vi "reallocate_pixel_mapper_arrays.vi"(7 "New pixels per spiral":T1=1 min=1 max=90000 step=1, 8 "error in":errorcluster, 9 "New image size":T2=128 items=["128x128 px"=128, "256x256 px"=256, "512x512 px"=512], 10 "Lookup arrays in":T3, 11 "Pixelhits array in":refnum<data-value>) -> (0 "error out":errorcluster, 2 "Lookup arrays out":T3, 3 "Pixelhits array out":refnum<data-value>)   [LabVIEW 2011, in "Fiberscope_library.lvlib"]
uses:
  Fiberscope_library.lvlib
  typedefs/lookup_arrays_ref_cluster.ctl
  typedefs/image_size_I32.ctl
  typedefs/pixel_per_spiral_I32.ctl
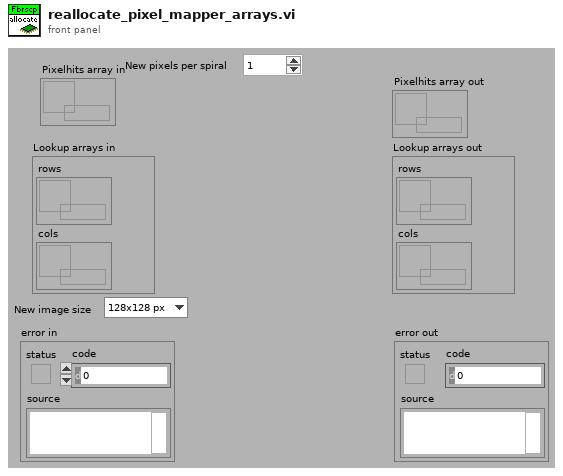
[diagram p1: front panel]
types:
  T1 = typedef "Fiberscope_library.lvlib/pixel_per_spiral_I32.ctl" = i32
  T2 = typedef "Fiberscope_library.lvlib/image_size_I32.ctl" = i32
  T3 = typedef "Fiberscope_library.lvlib/lookup_arrays_ref_cluster.ctl" = cluster{"rows":refnum<data-value>, "cols":refnum<data-value>}
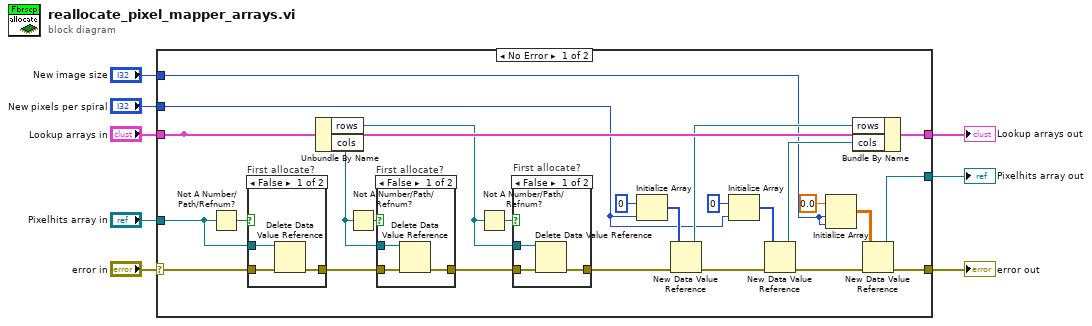
[diagram p0: block diagram]
diagram:
  n1 = case shown="No Error" "error in" {
    selector: "error in" -> [w26 w49]
    tunnel: [w19 w49] -> w7
    tunnel: [w17 w48] -> w4
    tunnel: "Pixelhits array in" -> [w16 w48]
    tunnel: [w27 w47] -> w3
    tunnel: "Lookup arrays in" -> [w28 w47]
    tunnel: "New image size" -> [w10 _]
    tunnel: "New pixels per spiral" -> [w9 _]
    frame No Error {
      n2 = Not A Number/Path/Refnum?(number/path/refnum=w16) -> (NaN/Path/Refnum?=w15:bool)
      n3 = case "First allocate?" shown="False" w15 {
        tunnel: w26 -> [w45 w46]
        tunnel: [w44 w46] -> w25
        tunnel: w16 -> [w43 _]
        frame False {
          n4 = Delete Data Value Reference(data value reference=w43, error in=w45) -> (error out=w44:errorcluster)  [unwired: 1 out]
        }
        frame True {
        }
      }
      n5 = Unbundle By Name(w28) -> ("rows"=w12:refnum<data-value>, "cols"=w14:refnum<data-value>)
      n6 = Not A Number/Path/Refnum?(number/path/refnum=w14) -> (NaN/Path/Refnum?=w13:bool)
      n7 = case "First allocate?" shown="False" w13 {
        tunnel: w14 -> [w41 _]
        tunnel: [w40 w42] -> w34
        tunnel: w25 -> [w39 w42]
        frame False {
          n8 = Delete Data Value Reference(data value reference=w41, error in=w39) -> (error out=w40:errorcluster)  [unwired: 1 out]
        }
        frame True {
        }
      }
      n9 = Not A Number/Path/Refnum?(number/path/refnum=w12) -> (NaN/Path/Refnum?=w11:bool)
      n10 = case "First allocate?" shown="False" w11 {
        tunnel: w34 -> [w37 w38]
        tunnel: w12 -> [w36 _]
        tunnel: [w35 w38] -> w24
        frame False {
          n11 = Delete Data Value Reference(data value reference=w36, error in=w37) -> (error out=w35:errorcluster)  [unwired: 1 out]
        }
        frame True {
        }
      }
      n12 = Initialize Array(0, w9) -> (w32:i32[])
      n13 = New Data Value Reference(data value=w32, error in=w24) -> (data value reference=w23:refnum<data-value>, error out=w30:errorcluster)
      n14 = Initialize Array(0, w9) -> (w31:i32[])
      n15 = New Data Value Reference(data value=w31, error in=w30) -> (data value reference=w22:refnum<data-value>, error out=w20:errorcluster)
      n16 = Initialize Array(0.0 ("element"), w10, w10) -> (w18:dbl[][])
      n17 = Bundle By Name(cluster=w28, "rows"=w23, "cols"=w22) -> (w27:T3)
      n18 = New Data Value Reference(data value=w18, error in=w20) -> (data value reference=w17:refnum<data-value>, error out=w19:errorcluster)
    }
    frame Error {
    }
  }
  "error out" <- w7
  "Lookup arrays out" <- w3
  "Pixelhits array out" <- w4
